vi "GPO_MODE - Type.vi"(8 "error in (no error)":errorcluster, 11 "GPO_MODE":T1) -> (0 "error out":errorcluster, 3 "GPO_MODE_VALUE":i32)   [LabVIEW 2015]
doc: "<b>GPO port state options</b>\nOFF : Output off.\nON : Logical level.\nFRAME_ACTIVE : High during exposure(integration) time + readout time + data transfer time.\nFRAME_ACTIVE_NEG : Low during exposure(integration) time + readout time + data trasnfer time.\nEXPOSURE_ACTIVE : High during exposure(integration) time.\nEXPOSURE_ACTIVE_NEG : Low during exposure(integration) time."
uses:
  C:/GIT/Cameras3.x/Integrations/Labview/xiLib/xiLIB_32bit/xiLIB/xiCamLib/API/x86/xiApi.NET.dll
  xiLIB_32bit/xiLIB/xiCamLib/API/x86/xiApi.NET.dll
  GPO_MODE.ctl
panel:
  # "Description: Defines GPO functionality.\nType: Integer.\nDefault: TRG_OFF\nPossible values:\nvalue\tmeaning\nXI_GPO_OFF**\tOutput is off (zero voltage or switched_off)\nXI_GPO_ON**\tOutput is on (voltage or switched_on)\nXI_GPO_FRAME_ACTIVE*\tOutput is on while frame exposure,read,transfer\nXI_GPO_FRAME_ACTIVE_NEG*\tOutput is off while frame exposure,read,transfer\nXI_GPO_EXPOSURE_ACTIVE*\tOutput is on while frame exposure\nXI_GPO_EXPOSURE_ACTIVE_NEG*\tOutput is off while frame exposure\n*Note1: Modes FRAME_ACTIVE or EXPOSURE_ACTIVE are supported only if XI_PRM_TRG_SOURCE is set to XI_TRG_SOFTWARE or XI_TRG_EDGE_RISING or XI_TRG_EDGE_FALLING. See section TriggerSource\n**Note2: Some camera families (e.g. MR) does not support the software control of outputs. Only one of mode: FRAME_ACTIVE and EXPOSURE_ACTIVE can be set."
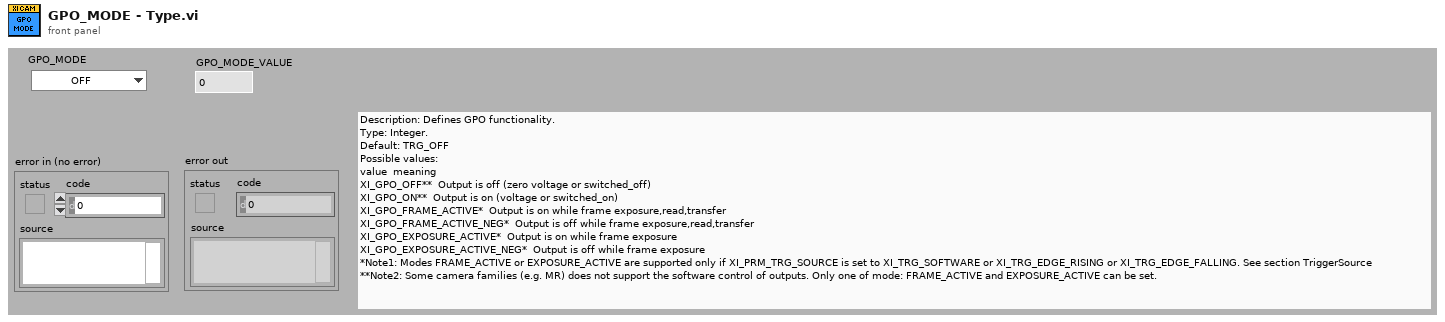
[diagram p1: front panel]
types:
  T1 = typedef "GPO_MODE.ctl" = enum16{"OFF", "ON", "FRAME_ACTIVE", "FRAME_ACTIVE_NEG", "EXPOSURE_ACTIVE", "EXPOSURE_ACTIVE_NEG"}
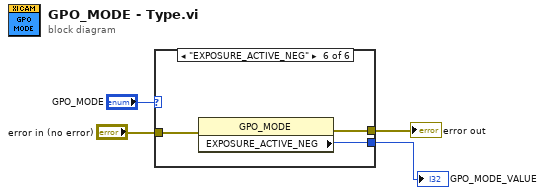
[diagram p0: block diagram]
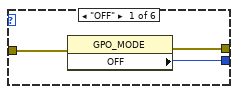
[diagram p2: hidden frame]
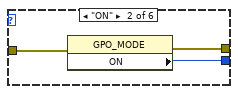
[diagram p3: hidden frame]
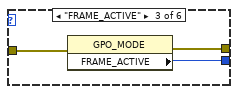
[diagram p4: hidden frame]
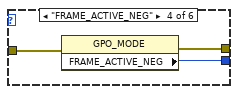
[diagram p5: hidden frame]
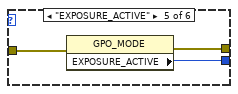
[diagram p6: hidden frame]
diagram:
  n1 = case shown="\"EXPOSURE_ACTIVE_NEG\"" "GPO_MODE" {
    tunnel: "error in (no error)" -> [w7 w10 w13 w16 w19 w22]
    tunnel: [w6 w9 w12 w15 w18 w21] -> w2
    tunnel: [w5 w8 w11 w14 w17 w20] -> w1
    frame "OFF" {
      n2 = property class="GPO_MODE"(error in=w7) -> (error out=w6:errorcluster, "OFF"=w5:i32)  [unwired: 1 in, 1 out]
    }
    frame "ON" {
      n3 = property class="GPO_MODE"(error in=w10) -> (error out=w9:errorcluster, "ON"=w8:i32)  [unwired: 1 in, 1 out]
    }
    frame "FRAME_ACTIVE" {
      n4 = property class="GPO_MODE"(error in=w13) -> (error out=w12:errorcluster, "FRAME_ACTIVE"=w11:i32)  [unwired: 1 in, 1 out]
    }
    frame "FRAME_ACTIVE_NEG" {
      n5 = property class="GPO_MODE"(error in=w16) -> (error out=w15:errorcluster, "FRAME_ACTIVE_NEG"=w14:i32)  [unwired: 1 in, 1 out]
    }
    frame "EXPOSURE_ACTIVE" {
      n6 = property class="GPO_MODE"(error in=w19) -> (error out=w18:errorcluster, "EXPOSURE_ACTIVE"=w17:i32)  [unwired: 1 in, 1 out]
    }
    frame "EXPOSURE_ACTIVE_NEG" {
      n7 = property class="GPO_MODE"(error in=w22) -> (error out=w21:errorcluster, "EXPOSURE_ACTIVE_NEG"=w20:i32)  [unwired: 1 in, 1 out]
    }
  }
  "error out" <- w2
  "GPO_MODE_VALUE" <- w1
